vi "sent by stage QM.vi"(8 "error in (no error)":errorcluster, 10 "ProceedMessage":refnum<class "ProceedMessage.lvclass">, 11 "Cascade in":refnum<class "Cascade.lvclass">) -> (0 "error out":errorcluster, 2 "send by stage?":bool, 3 "Cascade out":refnum<class "Cascade.lvclass">)   [LabVIEW 2012, in "Cascade.lvclass"]
uses:
  Cascade.lvclass
  <vilib>/Distrio/Murmex/ProceedMessage/ProceedMessage.lvclass
  Cascade.lvclass/Cascade.ctl
  <vilib>/Distrio/Murmex/Message/Message.lvclass
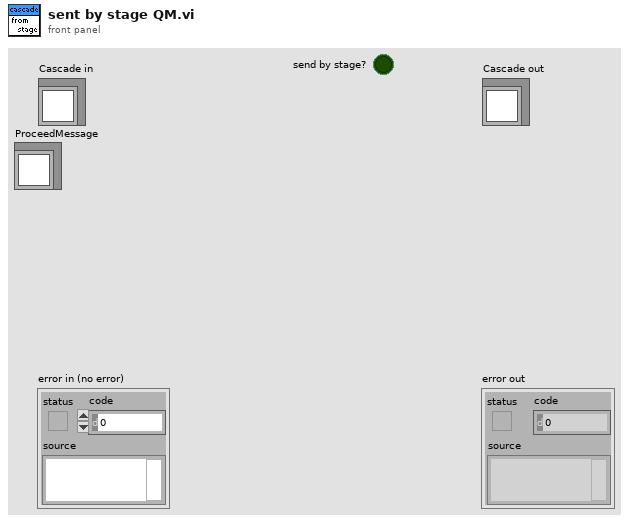
[diagram p1: front panel]
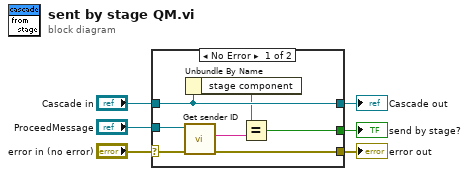
[diagram p0: block diagram]
diagram:
  n1 = case shown="No Error" "error in (no error)" {
    selector: "error in (no error)" -> [w13 w15]
    tunnel: [w12 w15] -> w5
    tunnel: [w10 w14] -> w3
    tunnel: "Cascade in" -> [w10 w14]
    tunnel: "ProceedMessage" -> [w11 _]
    tunnel: [w7 _] -> w1
    frame No Error {
      n2 = call <vilib>:"Get sender ID.vi"("error in (no error)"=w13, "Message in"=w11) -> ("error out"=w12:errorcluster, "sender"=w9:string)  [unwired: 7 in, 1 out]
      n3 = Unbundle By Name(w10) -> ("stage component"=w8:string)
      n4 = Equal?(x=w8, y=w9) -> (x = y?=w7:bool)
    }
    frame Error {
    }
  }
  "error out" <- w5
  "Cascade out" <- w3
  "send by stage?" <- w1
